vi "Popup Menu Get XY.vi"(0 "Vert Adj":i16, 2 "VI Ref":refnum<vi>, 7 "Str Ctrl Ref":refnum<vi>, 11 "Errror In":errorcluster) -> (8 "Screen Coordinates":T1, 15 "Error Out":errorcluster)   [LabVIEW 2020]
uses:
  <vilib>/Utility/miscctls.llb/LVPointTypeDef.ctl
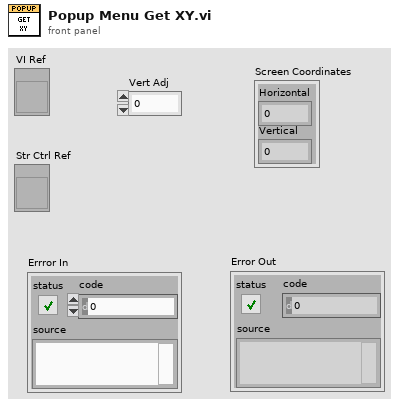
[diagram p1: front panel]
types:
  T1 = typedef "LVPointTypeDef.ctl" = cluster{"Horizontal":i16, "Vertical":i16}
  T2 = typedef "LVPositionTypeDef.ctl" = cluster{"Left":i32, "Top":i32}
  T3 = typedef "LVRectTypeDef.ctl" = cluster{"Left":i16, "Top":i16, "Right":i16, "Bottom":i16}
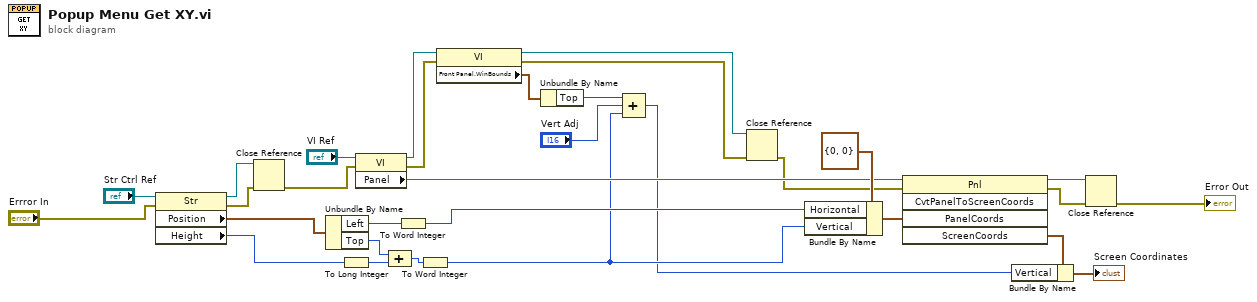
[diagram p0: block diagram]
diagram:
  n1 = property on="Property Node" class="Str"(reference="Str Ctrl Ref", error in="Errror In") -> (reference out=w18:refnum<vi>, error out=w16:errorcluster, "Position"=w23:T2, "Height"=w27:u32)
  n2 = Close Reference(reference=w18, error in (no error)=w16) -> (error out=w15:errorcluster)
  n3 = Unbundle By Name(w23) -> ("Left"=w29:i32, "Top"=w24:i32)
  n4 = To Long Integer(number=w27) -> (32bit integer=w26:i32)
  n5 = property class="VI"(reference="VI Ref", error in=w15) -> (reference out=w8:refnum<vi>, error out=w7:errorcluster, "Panel"=w21:refnum<vi>)
  n6 = Compound Arithmetic op=ADD(w24, w26) -> (w25:i32)
  n7 = To Word Integer(number=w29) -> (16bit integer=w28:i16)
  n8 = To Word Integer(number=w25) -> (16bit integer=w2:i16)
  n9 = property class="VI"(reference=w8, error in=w7) -> (reference out=w5:refnum<vi>, error out=w6:errorcluster, "Front Panel.WinBounds"=w11:T3)
  n10 = Unbundle By Name(w11) -> ("Top"=w4:i16)
  n11 = Compound Arithmetic op=ADD(w4, "Vert Adj", w2) -> (w1:i16)
  n12 = Close Reference(reference=w5, error in (no error)=w6) -> (error out=w14:errorcluster)
  n13 = Bundle By Name(cluster=T1 {"Horizontal"=0, "Vertical"=0} ("Panel Coordinates"), "Horizontal"=w28, "Vertical"=w2) -> (w30:T1)
  n14 = invoke class="Pnl" method="CvtPanelToScreenCoords"(reference=w21, error in=w14, "PanelCoords"=w30) -> (reference out=w19:refnum<vi>, error out=w13:errorcluster, "ScreenCoords"=w10:T1)  [unwired: 2 in, 2 out]
  n15 = Bundle By Name(cluster=w10, "Vertical"=w1) -> (→"Screen Coordinates":T1)
  n16 = Close Reference(reference=w19, error in (no error)=w13) -> (error out=→"Error Out":errorcluster)
